vi "test_TrajectoryAK101022Resonance.vi"() -> ()   [LabVIEW 2010, in "TrajectoryAK101022Resonance.lvclass"]
uses:
  TrajectoryAK101022Resonance.lvclass
  common/classes/SpaceVector/SpaceVector/SpaceVector.lvclass
  main/labview_source/type_definitions/enumerations/run_mode_enum.ctl
panel:
  out "last event":string
  in  "step size":dbl[unit]=4.9999999999999996e-06
  in  "repetitions":i32=-1 caption="repetitions (averagings per frame for stack, no. of volumes for fast volume scan )"
  in  "number of planes":i32=60
  in  "button:define":bool
  out "iterations per pixel":u16
  in  "pixel dwell time":dbl[unit]=1.5e-07 min=0.0 step=1e-08
  in  "y resolution":i32=100
  in  "createButton":bool
  in  "run button":bool
  in  "stop":bool
  in  "repetition rate":dbl[unit]=77.66990291262135
  in  "x resolution":i32=100
  in  "modify":bool
  in  "configure":bool
  in  "zoom":dbl(slide)=0.6603773584905661 scale=1.0..10.0
  # "Test VI for TrajectoryAK101022Resonance"
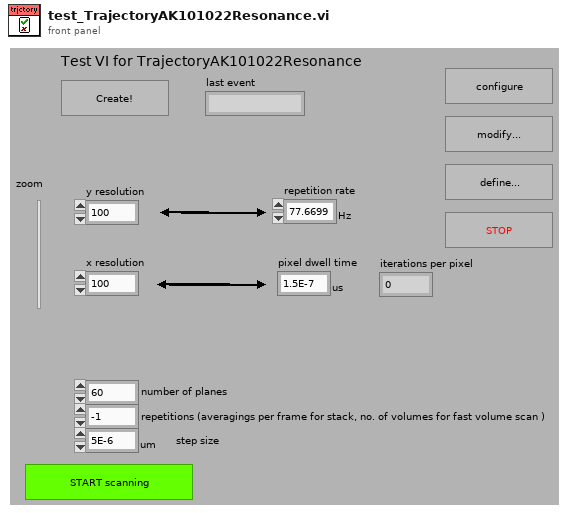
[diagram p1: front panel]
types:
  T1 = enum8{"Enabled", "Disabled", "Disabled and Grayed Out"}
  T2 = typedef "run_mode_enum.ctl" = enum16{"focus mode", "single sweep mode", "experiment mode"}
  T3 = typedef "plugin_specification.ctl" = cluster{"class path":string, "configuration":string, "label":string, "settings name":string}
  T4 = typedef "XComponentSpecification.xctl/data.ctl" = cluster{"class path":string, "configuration":string, "label":string, "settings name":string}
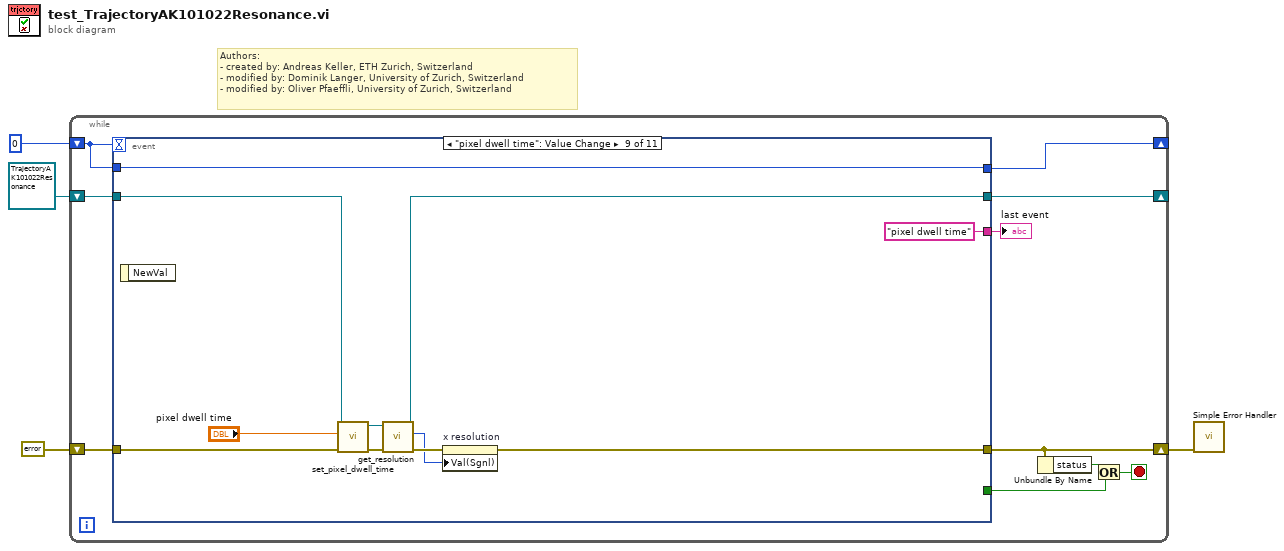
[diagram p0: block diagram]
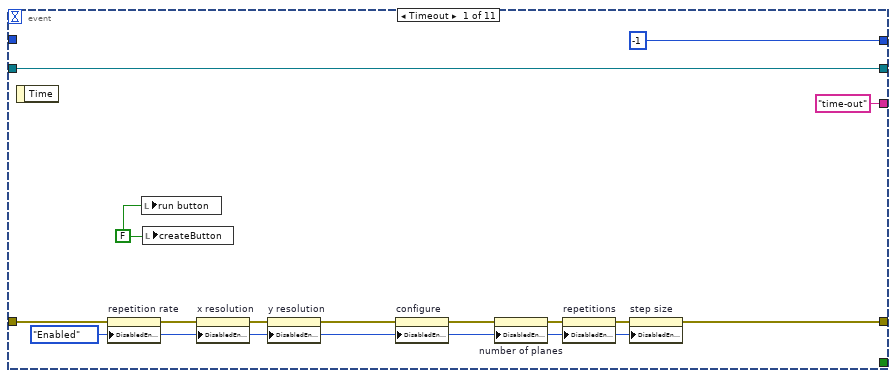
[diagram p2: hidden frame]
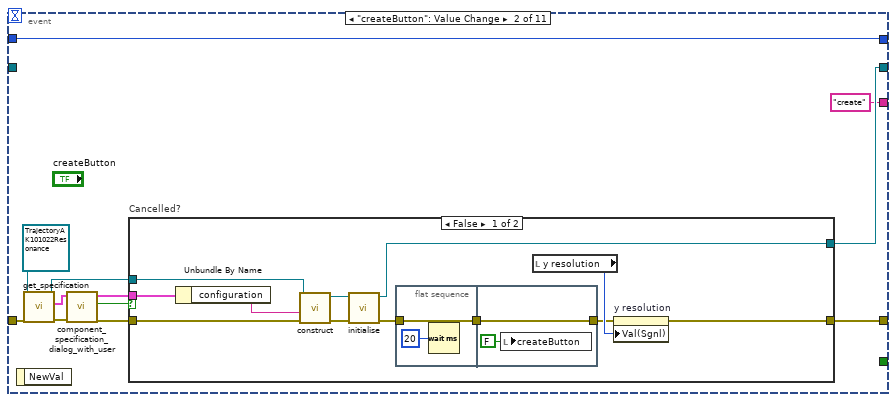
[diagram p3: hidden frame]
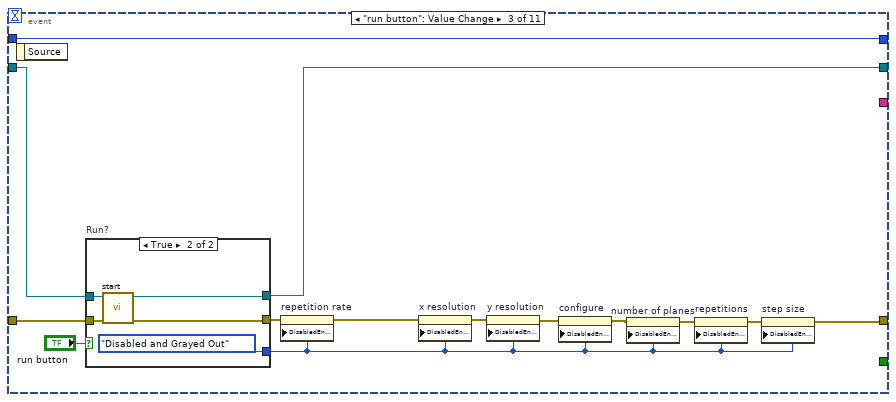
[diagram p5: hidden frame]
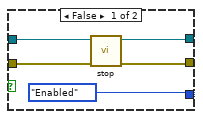
[diagram p6: hidden frame]
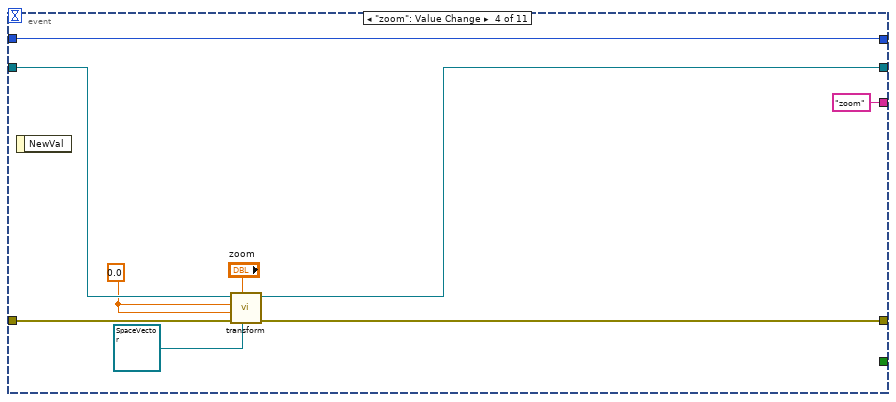
[diagram p7: hidden frame]
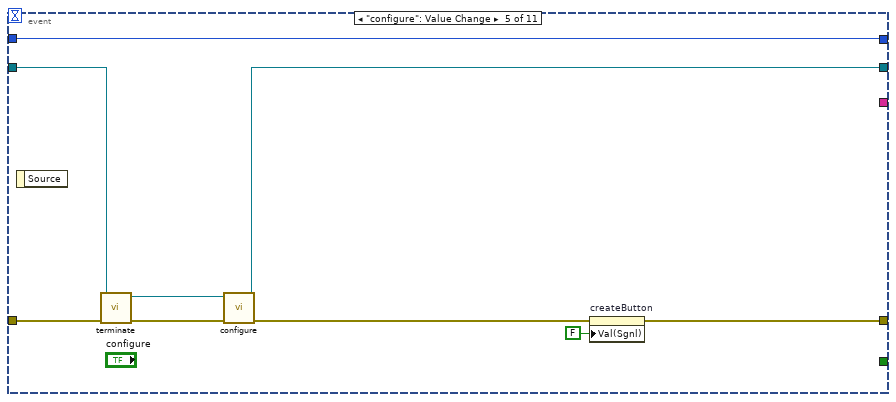
[diagram p8: hidden frame]
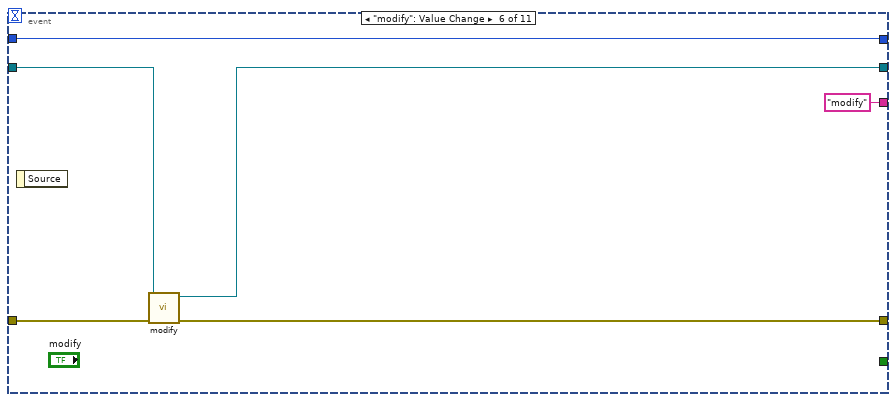
[diagram p9: hidden frame]
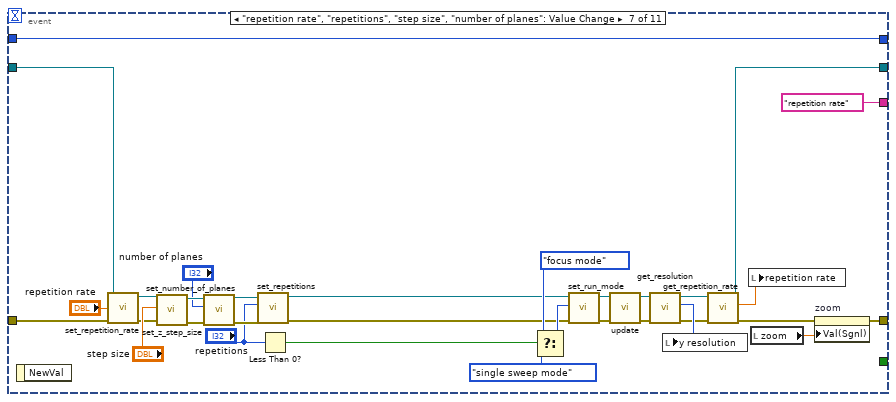
[diagram p10: hidden frame]
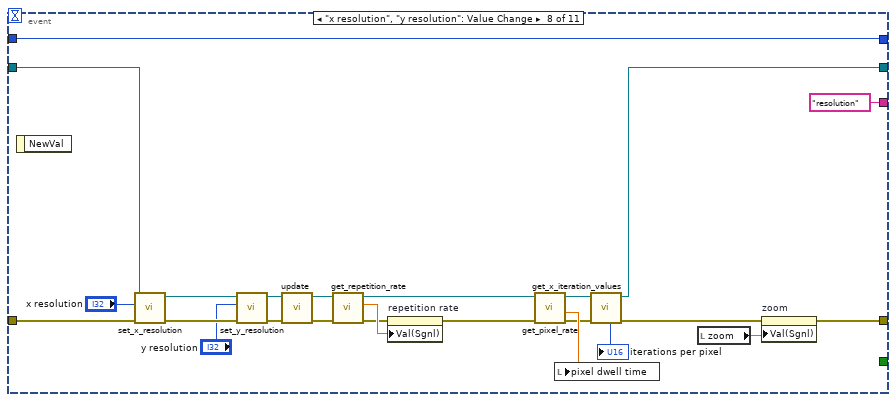
[diagram p11: hidden frame]
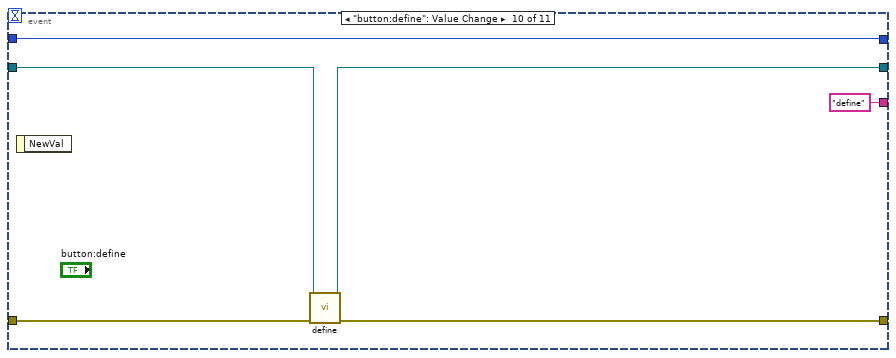
[diagram p12: hidden frame]
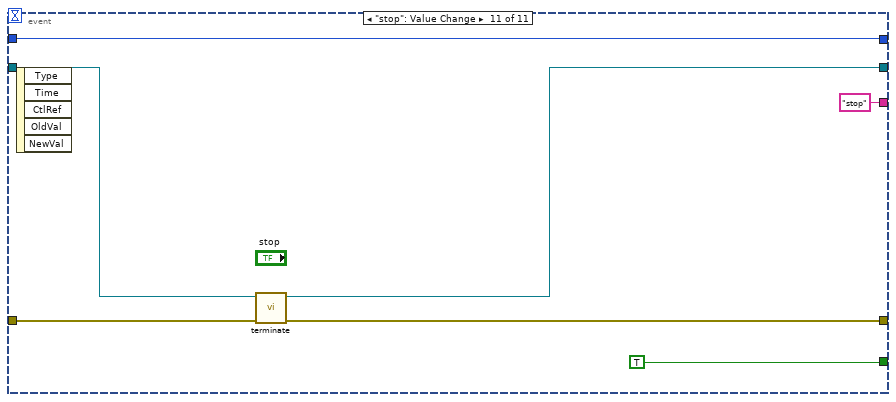
[diagram p13: hidden frame]
diagram:
  # "Authors: \n- created by: Andreas Keller, ETH Zurich, Switzerland\n- modified by: Dominik Langer, University of Zurich, Switzerland\n- modified by: Oliver Pfaeffli, University of Zurich, Switzerland"
  n1 = while {
    shift-right: [w12] -> _
    shift-left: refnum<class "TrajectoryAK101022Resonance.lvclass"> refnum ("TrajectoryAK101022Resonance.lvclass") -> [w11]
    shift-right: [w9] -> w3
    shift-left: errorcluster {"status"=FALSE, "code"=0, "source"=""} ("error out") -> [w10]
    shift-right: [w6] -> _
    shift-left: 0 -> [w7]
    stop <- w13 stop-if-true
    n2 = event shown="[8] \"pixel dwell time\": Value Change" {
      selector: _ -> [_ _ _ _ _ _ _ _ _ _ _]
      dyn-events: _ -> [_ _ _ _ _ _ _ _ _ _ _]
      timeout: w7 -> [_ _ _ _ _ _ _ _ _ _ _]
      tunnel: [w16 w37 w59 w84 w92 w102 w130 w153 w164 w176 w180] -> w9
      tunnel: w10 -> [w24 w34 w69 w89 w96 w104 w135 w161 w171 w177 w181]
      tunnel: [w22 w39 w68 w83 w91 w101 w126 w142 w166 w174 w182] -> w12
      tunnel: w11 -> [w22 _ w70 w90 w98 w105 w136 w160 w170 w175 w183]
      tunnel: [_ _ _ _ _ _ _ _ _ _ TRUE] -> w8
      tunnel: w7 -> [_ w38 w67 w87 w99 w103 w134 w159 w172 w178 w184]
      tunnel: [-1 w38 w67 w87 w99 w103 w134 w159 w172 w178 w184] -> w6
      tunnel: ["time-out" "create" _ "zoom" _ "modify" "repetition rate" "resolution" "pixel dwell time" "define" "stop"] -> w5
      event Timeout {
        w18 = T1."Enabled" ("Disabled")
        w23 = FALSE ("createButton")
        n3 = event-data() -> ()  [unwired: 1 in, 1 out]
        n4 = property on="repetition rate" class="DigNum (strict)"(error in=w24, "DisabledEnum"=w18) -> (error out=w21:errorcluster)  [unwired: 1 in, 1 out]
        n5 = local write "run button"(w23) -> ()
        n6 = local write "createButton"(w23) -> ()
        n7 = property on="x resolution" class="DigNum (strict)"(error in=w21, "DisabledEnum"=w18) -> (error out=w26:errorcluster)  [unwired: 1 in, 1 out]
        n8 = property on="y resolution" class="DigNum (strict)"(error in=w26, "DisabledEnum"=w18) -> (error out=w25:errorcluster)  [unwired: 1 in, 1 out]
        n9 = property on="configure" class="Bool"(error in=w25, "DisabledEnum"=w18) -> (error out=w17:errorcluster)  [unwired: 1 in, 1 out]
        n10 = property on="number of planes" class="DigNum (strict)"(error in=w17, "DisabledEnum"=w18) -> (error out=w20:errorcluster)  [unwired: 1 in, 1 out]
        n11 = property on="repetitions" class="DigNum (strict)"(error in=w20, "DisabledEnum"=w18) -> (error out=w19:errorcluster)  [unwired: 1 in, 1 out]
        n12 = property on="step size" class="DigNum (strict)"(error in=w19, "DisabledEnum"=w18) -> (error out=w16:errorcluster)  [unwired: 1 in, 1 out]
      }
      event "createButton": Value Change {
        n13 = event-data() -> ()  [unwired: 1 in, 1 out]
        n14 = call-dynamic "get_specification.vi"("error in (no error)"=w34, "GenericPlugin in"=refnum<class "TrajectoryAK101022Resonance.lvclass"> refnum ("TrajectoryAK101022Resonance.lvclass")) -> ("error out"=w36:errorcluster, "component specification"=w32:T3, "GenericPlugin out"=w35:refnum<class "TrajectoryAK101022Resonance.lvclass">)  [unwired: 6 in, 1 out]
        n15 = call "component_specification_dialog_with_user.vi"("error in (no error)"=w36, "component specification in"=w32) -> ("error out"=w33:errorcluster, "cancelled?"=w30:bool, "component specification out"=w31:T4)  [unwired: 7 in]
        n16 = case "Cancelled?" shown="False" w30 {
          tunnel: [w49 w56] -> w39
          tunnel: [w40 w57] -> w37
          tunnel: w35 -> [w47 w56]
          tunnel: w33 -> [w46 w57]
          tunnel: w31 -> [w45 _]
          frame False {
            n17 = Unbundle By Name(w45) -> ("configuration"=w44:string)
            n18 = call-dynamic "construct.vi"("error in (no error)"=w46, "configuration name"=w44, "GenericPlugin in"=w47) -> ("error out"=w51:errorcluster, "GenericPlugin out"=w50:refnum<class "TrajectoryAK101022Resonance.lvclass">)  [unwired: 7 in]
            n19 = call-dynamic "initialise.vi"("error in (no error)"=w51, "GenericPlugin in"=w50) -> ("error out"=w43:errorcluster, "GenericPlugin out"=w49:refnum<class "TrajectoryAK101022Resonance.lvclass">)  [unwired: 8 in]
            n20 = flat-sequence {
              tunnel: w43 -> [w53]
              tunnel: [w53] -> w41
              tunnel: [w55] -> w42
              tunnel: w41 -> [w55]
              frame #0 {
                n21 = Wait (ms)(milliseconds to wait=u32 20) -> ()  [unwired: 1 out]
              }
              frame #1 {
                n22 = local write "createButton"(FALSE ("createButton")) -> ()
              }
            }
            n23 = local read "y resolution"() -> (w48:i32)
            n24 = property on="y resolution" class="DigNum (strict)"(error in=w42, "Val(Sgnl)"=w48) -> (error out=w40:errorcluster)  [unwired: 1 in, 1 out]
          }
          frame True {
          }
        }
      }
      event "run button": Value Change {
        n25 = event-data() -> ()  [unwired: 1 in, 1 out]
        n26 = case "Run?" shown="True" "run button" {
          tunnel: w70 -> [w73 w79]
          tunnel: w69 -> [w75 w80]
          tunnel: [w74 w78] -> w66
          tunnel: [w72 w77] -> w68
          tunnel: [T1."Enabled" ("Disabled") T1."Disabled and Grayed Out" ("Disabled")] -> w58
          frame False {
            n27 = call-dynamic "stop.vi"("error in (no error)"=w75, "TrajectoryMG100122GenericFPGA in"=w73) -> ("error out"=w74:errorcluster, "TrajectoryMG100122GenericFPGA out"=w72:refnum<class "TrajectoryAK101022Resonance.lvclass">)  [unwired: 8 in]
          }
          frame True {
            n28 = call-dynamic "start.vi"("error in (no error)"=w80, "TrajectoryMG100122GenericFPGA in"=w79) -> ("error out"=w78:errorcluster, "TrajectoryMG100122GenericFPGA out"=w77:refnum<class "TrajectoryAK101022Resonance.lvclass">)  [unwired: 8 in]
          }
        }
        n29 = property on="repetition rate" class="DigNum (strict)"(error in=w66, "DisabledEnum"=w58) -> (error out=w63:errorcluster)  [unwired: 1 in, 1 out]
        n30 = property on="x resolution" class="DigNum (strict)"(error in=w63, "DisabledEnum"=w58) -> (error out=w65:errorcluster)  [unwired: 1 in, 1 out]
        n31 = property on="y resolution" class="DigNum (strict)"(error in=w65, "DisabledEnum"=w58) -> (error out=w64:errorcluster)  [unwired: 1 in, 1 out]
        n32 = property on="configure" class="Bool"(error in=w64, "DisabledEnum"=w58) -> (error out=w62:errorcluster)  [unwired: 1 in, 1 out]
        n33 = property on="number of planes" class="DigNum (strict)"(error in=w62, "DisabledEnum"=w58) -> (error out=w61:errorcluster)  [unwired: 1 in, 1 out]
        n34 = property on="repetitions" class="DigNum (strict)"(error in=w61, "DisabledEnum"=w58) -> (error out=w60:errorcluster)  [unwired: 1 in, 1 out]
        n35 = property on="step size" class="DigNum (strict)"(error in=w60, "DisabledEnum"=w58) -> (error out=w59:errorcluster)  [unwired: 1 in, 1 out]
      }
      event "zoom": Value Change {
        w86 = dbl[unit] 0.0 ("z angle (phi)")
        n36 = event-data() -> ()  [unwired: 1 in, 1 out]
        n37 = call-dynamic "transform.vi"("offset"=refnum<class "SpaceVector.lvclass"> refnum, "zoom"="zoom", "error in (no error)"=w89, "x angle (psi)"=w86, "z angle (phi)"=w86, "TrajectoryAK101022Resonance in"=w90) -> ("error out"=w84:errorcluster, "TrajectoryAK101022Resonance out"=w83:refnum<class "TrajectoryAK101022Resonance.lvclass">)  [unwired: 4 in]
      }
      event "configure": Value Change {
        n38 = event-data() -> ()  [unwired: 1 in, 1 out]
        n39 = call-dynamic "terminate.vi"("error in (no error)"=w96, "GenericPlugin in"=w98) -> ("error out"=w95:errorcluster, "GenericPlugin out"=w97:refnum<class "TrajectoryAK101022Resonance.lvclass">)  [unwired: 8 in]
        n40 = call-dynamic "configure.vi"("error in (no error)"=w95, "GenericPlugin in"=w97) -> ("error out"=w93:errorcluster, "GenericPlugin out"=w91:refnum<class "TrajectoryAK101022Resonance.lvclass">)  [unwired: 8 in]
        n41 = property on="createButton" class="Bool (strict)"(error in=w93, "Val(Sgnl)"=FALSE ("Value (Signaling)")) -> (error out=w92:errorcluster)  [unwired: 1 in, 1 out]
      }
      event "modify": Value Change {
        n42 = event-data() -> ()  [unwired: 1 in, 1 out]
        n43 = call-dynamic "modify.vi"("error in (no error)"=w104, "TrajectoryAK101022Resonance in"=w105) -> ("error out"=w102:errorcluster, "TrajectoryAK101022Resonance out"=w101:refnum<class "TrajectoryAK101022Resonance.lvclass">)  [unwired: 8 in]
      }
      event "repetition rate", "repetitions", "step size", "number of planes": Value Change {
        n44 = event-data() -> ()  [unwired: 1 in, 1 out]
        n45 = call-dynamic "set_repetition_rate.vi"("error in (no error)"=w135, "repetition rate"="repetition rate", "TrajectoryAK101022Resonance in"=w136) -> ("error out"=w111:errorcluster, "TrajectoryAK101022Resonance out"=w110:refnum<class "TrajectoryAK101022Resonance.lvclass">)  [unwired: 7 in]
        n46 = call-dynamic "set_z_step_size.vi"("error in (no error)"=w111, "z step size"="step size", "TrajectoryAK101022Resonance in"=w110) -> ("error out"=w114:errorcluster, "TrajectoryAK101022Resonance out"=w117:refnum<class "TrajectoryAK101022Resonance.lvclass">)  [unwired: 7 in]
        n47 = call-dynamic "set_number_of_planes.vi"("error in (no error)"=w114, "Number of planes"="number of planes", "TrajectoryAK101022Resonance in"=w117) -> ("error out"=w112:errorcluster, "TrajectoryAK101022Resonance out"=w113:refnum<class "TrajectoryAK101022Resonance.lvclass">)  [unwired: 7 in]
        n48 = call-dynamic "set_repetitions.vi"("error in (no error)"=w112, "repetitions"="repetitions", "GenericTrajectory in"=w113) -> ("error out"=w107:errorcluster, "GenericTrajectory out"=w106:refnum<class "TrajectoryAK101022Resonance.lvclass">)  [unwired: 7 in]
        n49 = Less Than 0?(x="repetitions") -> (x < 0?=w121:bool)
        n50 = Select(t=run_mode_enum."focus mode", s=w121, f=run_mode_enum."single sweep mode" ("run mode")) -> (s? t:f=w119:T2)
        n51 = call-dynamic "set_run_mode.vi"("error in (no error)"=w107, "run mode"=w119, "GenericPlugin in"=w106) -> ("error out"=w123:errorcluster, "GenericPlugin out"=w122:refnum<class "TrajectoryAK101022Resonance.lvclass">)  [unwired: 7 in]
        n52 = call-dynamic "update.vi"("error in (no error)"=w123, "TrajectoryAK101022Resonance in"=w122) -> ("error out"=w133:errorcluster, "TrajectoryAK101022Resonance out"=w132:refnum<class "TrajectoryAK101022Resonance.lvclass">)  [unwired: 8 in]
        n53 = call-dynamic "get_resolution.vi"("error in (no error)"=w133, "TrajectoryAK101022Resonance in"=w132) -> ("error out"=w125:errorcluster, "y resolution"=w128:i32, "TrajectoryAK101022Resonance out"=w124:refnum<class "TrajectoryAK101022Resonance.lvclass">)  [unwired: 6 in, 1 out]
        n54 = local write "y resolution"(w128) -> ()
        n55 = call-dynamic "get_repetition_rate.vi"("error in (no error)"=w125, "GenericTrajectory in"=w124) -> ("error out"=w127:errorcluster, "repetition rate"=w129:dbl[unit], "GenericTrajectory out"=w126:refnum<class "TrajectoryAK101022Resonance.lvclass">)  [unwired: 7 in]
        n56 = local write "repetition rate"(w129) -> ()
        n57 = local read "zoom"() -> (w131:dbl)
        n58 = property on="zoom" class="Slide (strict)"(error in=w127, "Val(Sgnl)"=w131) -> (error out=w130:errorcluster)  [unwired: 1 in, 1 out]
      }
      event "x resolution", "y resolution": Value Change {
        n59 = event-data() -> ()  [unwired: 1 in, 1 out]
        n60 = call-dynamic "set_x_resolution.vi"("error in (no error)"=w161, "x resolution"="x resolution", "TrajectoryAK101022Resonance in"=w160) -> ("error out"=w158:errorcluster, "TrajectoryAK101022Resonance out"=w156:refnum<class "TrajectoryAK101022Resonance.lvclass">)  [unwired: 7 in]
        n61 = call-dynamic "set_y_resolution.vi"("error in (no error)"=w158, "y resolution"="y resolution", "TrajectoryAK101022Resonance in"=w156) -> ("error out"=w155:errorcluster, "TrajectoryAK101022Resonance out"=w157:refnum<class "TrajectoryAK101022Resonance.lvclass">)  [unwired: 7 in]
        n62 = call-dynamic "update.vi"("error in (no error)"=w155, "TrajectoryAK101022Resonance in"=w157) -> ("error out"=w151:errorcluster, "TrajectoryAK101022Resonance out"=w150:refnum<class "TrajectoryAK101022Resonance.lvclass">)  [unwired: 8 in]
        n63 = call-dynamic "get_repetition_rate.vi"("error in (no error)"=w151, "GenericTrajectory in"=w150) -> ("error out"=w139:errorcluster, "repetition rate"=w140:dbl[unit], "GenericTrajectory out"=w149:refnum<class "TrajectoryAK101022Resonance.lvclass">)  [unwired: 7 in]
        n64 = property on="repetition rate" class="DigNum (strict)"(error in=w139, "Val(Sgnl)"=w140) -> (error out=w138:errorcluster)  [unwired: 1 in, 1 out]
        n65 = call-dynamic "get_pixel_rate.vi"("error in (no error)"=w138, "TrajectoryAK101022Resonance in"=w149) -> ("error out"=w145:errorcluster, "pixel dwell time"=w148:dbl[unit], "TrajectoryAK101022Resonance out"=w143:refnum<class "TrajectoryAK101022Resonance.lvclass">)  [unwired: 6 in, 1 out]
        n66 = local write "pixel dwell time"(w148) -> ()
        n67 = call-dynamic "get_x_iteration_values.vi"("error in (no error)"=w145, "TrajectoryAK101022Resonance in"=w143) -> ("error out"=w144:errorcluster, "TrajectoryAK101022Resonance out"=w142:refnum<class "TrajectoryAK101022Resonance.lvclass">, "iterations per pixel"=→"iterations per pixel":u16)  [unwired: 4 in, 3 out]
        n68 = local read "zoom"() -> (w152:dbl)
        n69 = property on="zoom" class="Slide (strict)"(error in=w144, "Val(Sgnl)"=w152) -> (error out=w153:errorcluster)  [unwired: 1 in, 1 out]
      }
      event "pixel dwell time": Value Change {
        n70 = event-data() -> ()  [unwired: 1 in, 1 out]
        n71 = call-dynamic "set_pixel_dwell_time.vi"("error in (no error)"=w171, "pixel-dwell time"="pixel dwell time", "TrajectoryAK101022Resonance in"=w170) -> ("error out"=w168:errorcluster, "TrajectoryAK101022Resonance out"=w167:refnum<class "TrajectoryAK101022Resonance.lvclass">)  [unwired: 7 in]
        n72 = call-dynamic "get_resolution.vi"("error in (no error)"=w168, "TrajectoryAK101022Resonance in"=w167) -> ("error out"=w165:errorcluster, "x resolution"=w163:i32, "TrajectoryAK101022Resonance out"=w166:refnum<class "TrajectoryAK101022Resonance.lvclass">)  [unwired: 6 in, 1 out]
        n73 = property on="x resolution" class="DigNum (strict)"(error in=w165, "Val(Sgnl)"=w163) -> (error out=w164:errorcluster)  [unwired: 1 in, 1 out]
      }
      event "button:define": Value Change {
        n74 = event-data() -> ()  [unwired: 1 in, 1 out]
        n75 = call-dynamic "define.vi"("error in (no error)"=w177, "TrajectoryAK101022Resonance in"=w175) -> ("error out"=w176:errorcluster, "TrajectoryAK101022Resonance out"=w174:refnum<class "TrajectoryAK101022Resonance.lvclass">)  [unwired: 8 in]
      }
      event "stop": Value Change {
        n76 = event-data() -> ()  [unwired: 1 in, 5 out]
        n77 = call-dynamic "terminate.vi"("error in (no error)"=w181, "GenericPlugin in"=w183) -> ("error out"=w180:errorcluster, "GenericPlugin out"=w182:refnum<class "TrajectoryAK101022Resonance.lvclass">)  [unwired: 8 in]
      }
    }
    "last event" <- w5
    n78 = Unbundle By Name(w9) -> ("status"=w14:bool)
    n79 = Or(x=w14, y=w8) -> (x .or. y?=w13:bool)
  }
  n80 = call <vilib>:"Simple Error Handler.vi"("error in (no error)"=w3) -> ()  [unwired: 4 in, 5 out]
